vi "Command Pre-Buffer.vi"(2 "All Robot Commands In":T1, 3 "Startup":bool, 4 "Cmd Parameter 4":string, 5 "Cmd Parameter 3":dbl, 6 "Cmd Parameter 2":dbl, 7 "Cmd Parameter 1":dbl) -> (0 "All Robot Commands Out":T1, 1 "Completed":bool)   [LabVIEW 2016]
uses:
  Subsystems/All Robot Commands.ctl
  Subsystems/Drive and Climb SS/Drive + Climb Commands 2017.ctl
  Subsystems/Gear Delivery SS/Gear Delivery Commands.ctl
  Subsystems/Conveyor and Shooter SS/Conveyor and Shooter Commands.ctl
  Subsystems/Ball Intake SS/Ball Intake Commands.ctl
  Command Execution State.ctl
panel:
  # "Sample robot\ncontrol output.\nReplace with \nactual teleop \ncontrol signal \nstructure."
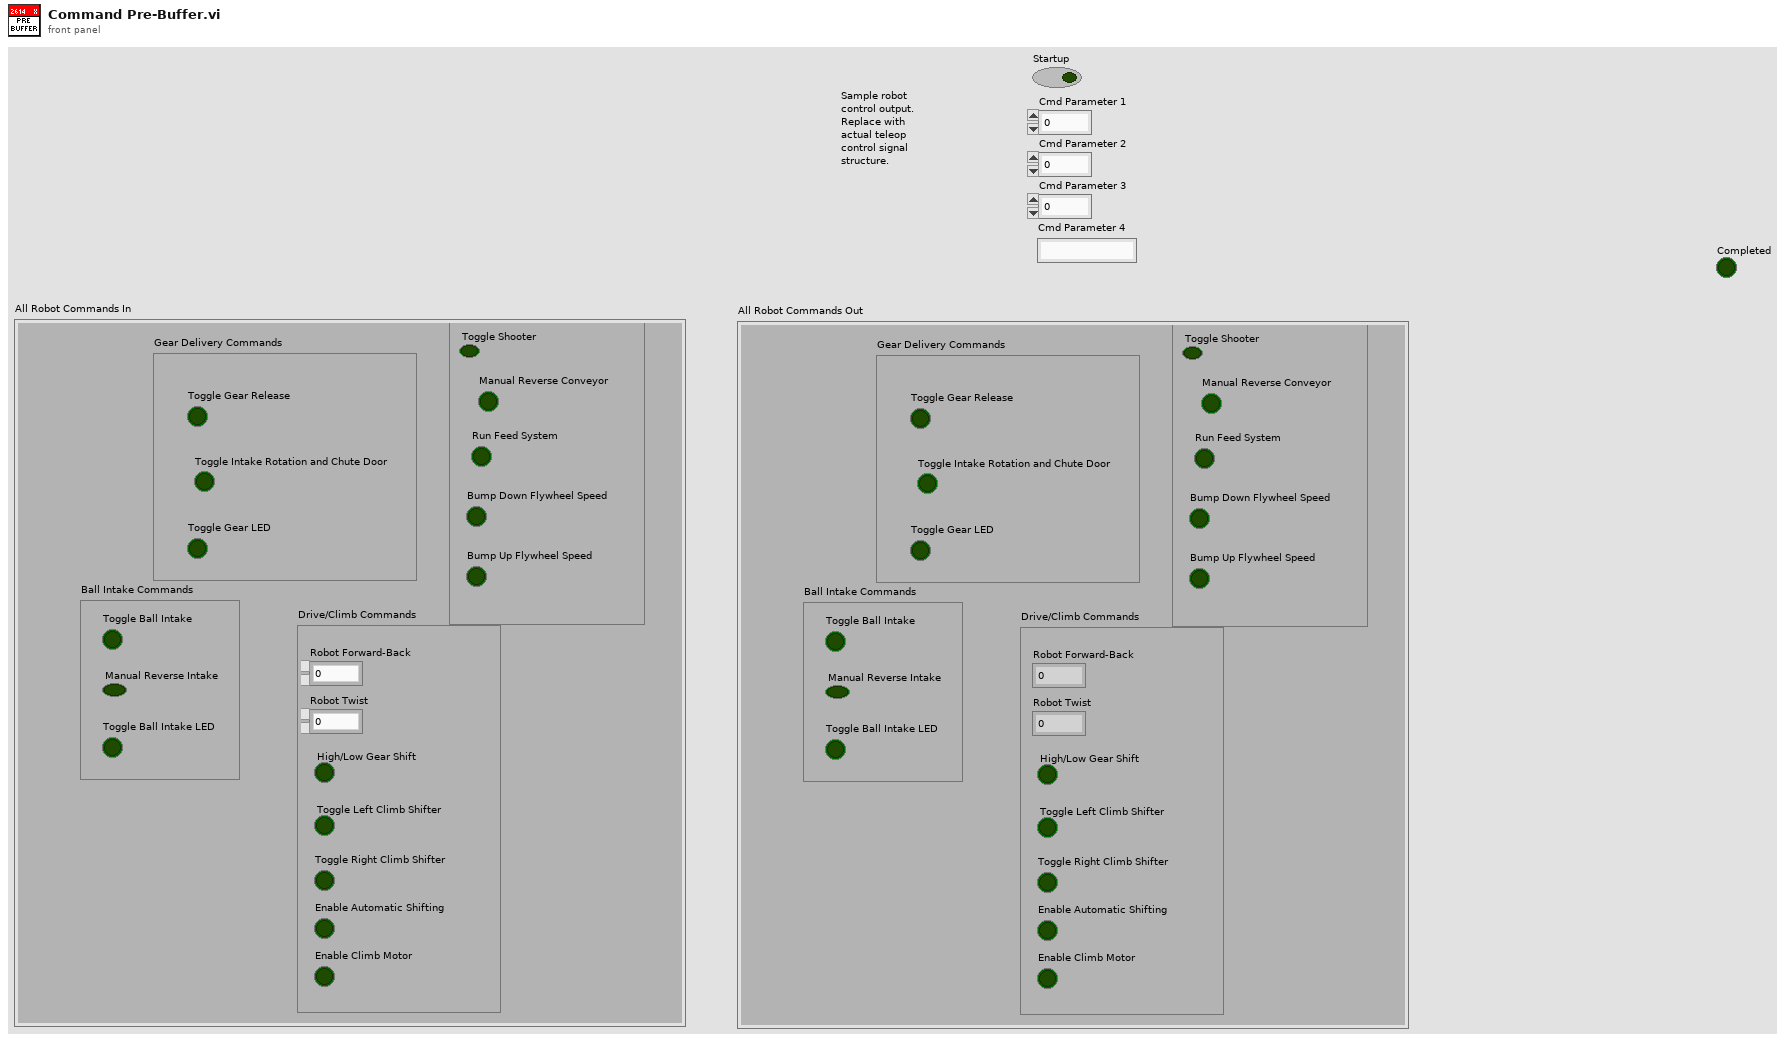
[diagram p1: front panel]
types:
  T1 = typedef "All Robot Commands.ctl" = cluster{"Drive/Climb Commands":T2, "Gear Delivery Commands":T3, "Shooter and Conveyor Commands":T4, "Ball Intake Commands":T5}
  T2 = typedef "Drive + Climb Commands 2017.ctl" = cluster{"Robot Forward-Back":dbl, "Robot Twist":dbl, "High/Low Gear Shift":bool, "Toggle Left Climb Shifter":bool, "Toggle Right Climb Shifter":bool, "Enable Automatic Shifting":bool, "Enable Climb Motor ":bool}
  T3 = typedef "Gear Delivery Commands.ctl" = cluster{"Toggle Gear Release":bool, "Toggle Intake Rotation and Chute Door":bool, "Toggle Gear LED":bool}
  T4 = typedef "Conveyor and Shooter Commands.ctl" = cluster{"Toggle Shooter":bool, "Manual Reverse Conveyor":bool, "Run Feed System":bool, "Bump Down Flywheel Speed":bool, "Bump Up Flywheel Speed":bool}
  T5 = typedef "Ball Intake Commands.ctl" = cluster{"Toggle Ball Intake":bool, "Manual Reverse Intake":bool, "Toggle Ball Intake LED":bool}
  T6 = typedef "Command Execution State.ctl" = enum16{"Initialize", "Execute", "Finish"}
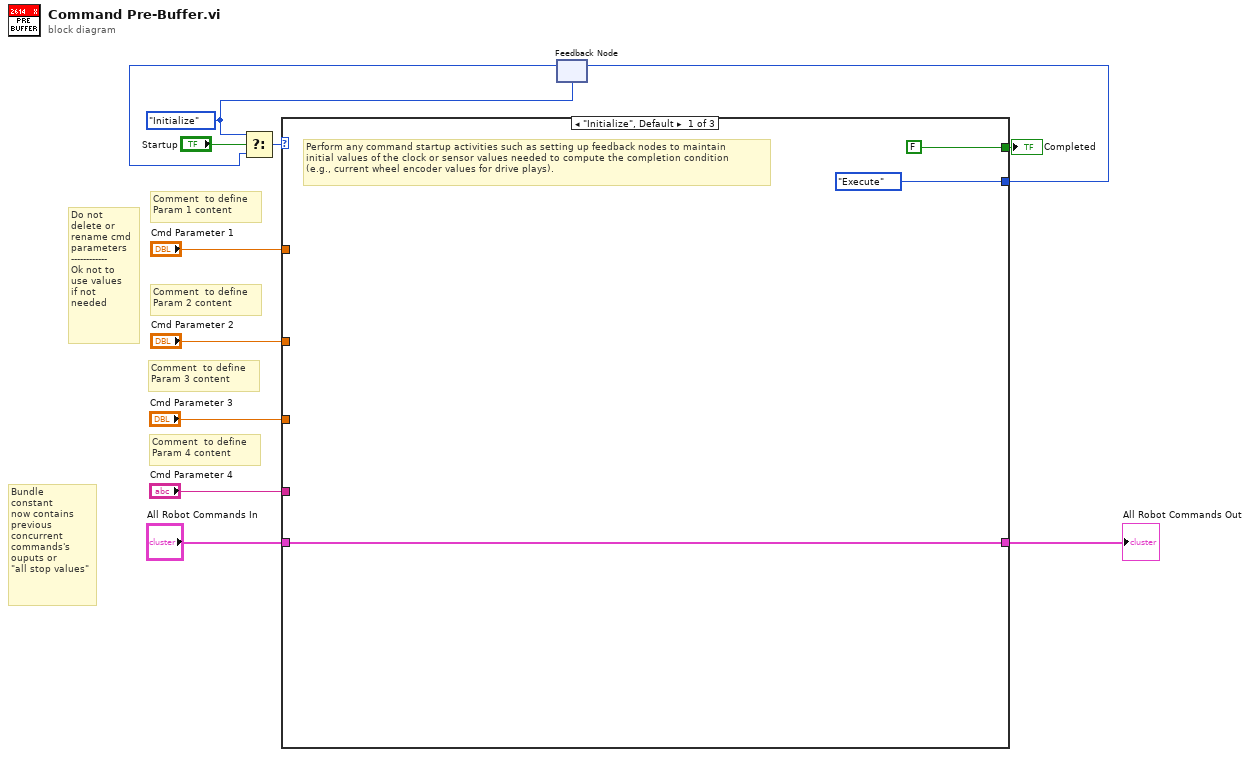
[diagram p0: block diagram]
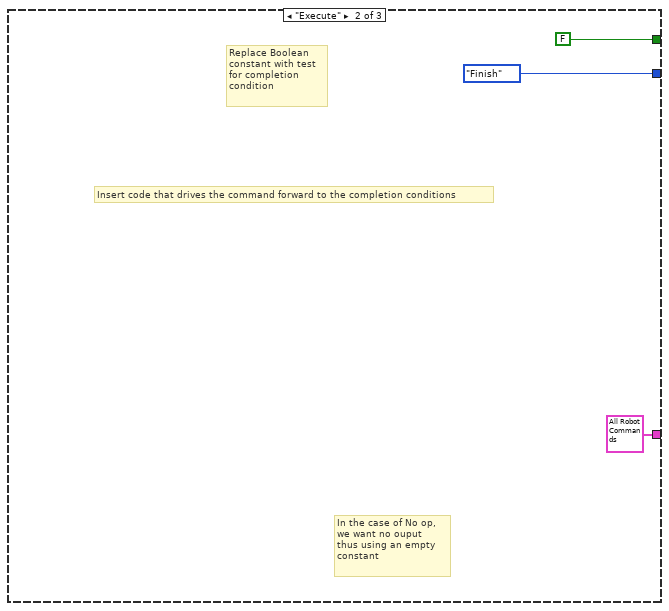
[diagram p2: hidden frame]
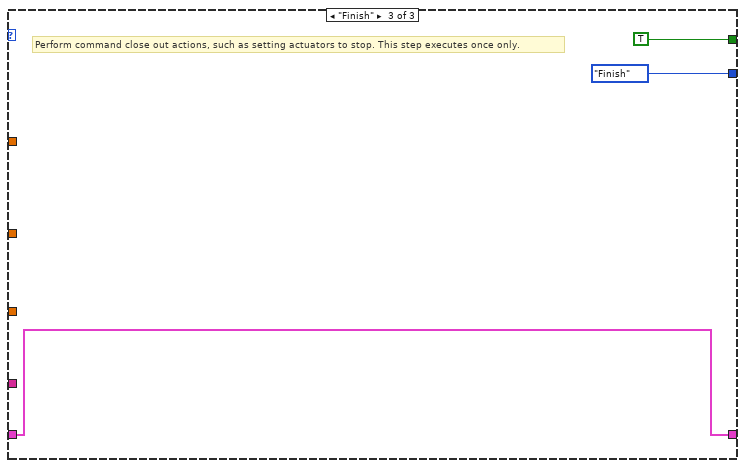
[diagram p3: hidden frame]
diagram:
  w7 = Command_Execution_State."Initialize" ("Play State")
  # "Comment  to define\nParam 4 content"
  # "Comment  to define\nParam 3 content"
  # "Bundle \nconstant\nnow contains\nprevious \nconcurrent\ncommands's\nouputs or\n\"all stop values\""
  # "Do not \ndelete or\nrename cmd\nparameters\n------------\nOk not to \nuse values\nif not \nneeded"
  # "Comment  to define\nParam 2 content"
  # "Comment  to define\nParam 1 content"
  n1 = feedback #1(w7) -> (w8:T6)
  n2 = Select(t=w7, s="Startup", f=w8) -> (s? t:f=w12:T6)
  n3 = case shown="\"Initialize\", Default" w12 {
    tunnel: [FALSE FALSE TRUE] -> w10
    tunnel: [Command_Execution_State."Execute" ("Play State") Command_Execution_State."Finish" ("Play State") Command_Execution_State."Finish" ("f")] -> w9
    tunnel: "Cmd Parameter 1" -> [_ _ _]
    tunnel: "Cmd Parameter 2" -> [_ _ _]
    tunnel: [w13 T1 {"Drive/Climb Commands"={"Robot Forward-Back"=0.0, "Robot Twist"=0.0, "High/Low Gear Shift"=FALSE, "Toggle Left Climb Shifter"=FALSE, "Toggle Right Climb Shifter"=FALSE, "Enable Automatic Shifting"=FALSE, "Enable Climb Motor "=FALSE}, "Gear Delivery Commands"={"Toggle Gear Release"=FALSE, "Toggle Intake Rotation and Chute Door"=FALSE, "Toggle Gear LED"=FALSE}, "Shooter and Conveyor Commands"={"Toggle Shooter"=FALSE, "Manual Reverse Conveyor"=FALSE, "Run Feed System"=FALSE, "Bump Down Flywheel Speed"=FALSE, "Bump Up Flywheel Speed"=FALSE}, "Ball Intake Commands"={"Toggle Ball Intake"=FALSE, "Manual Reverse Intake"=FALSE, "Toggle Ball Intake LED"=FALSE}} ("All Robot Commands") w19] -> w1
    tunnel: "All Robot Commands In" -> [w13 _ w19]
    tunnel: "Cmd Parameter 3" -> [_ _ _]
    tunnel: "Cmd Parameter 4" -> [_ _ _]
    frame "Initialize", Default {
      # "Perform any command startup activities such as setting up feedback nodes to maintain \ninitial values of the clock or sensor values needed to compute the completion condition\n(e.g., current wheel encoder values for drive plays)."
    }
    frame "Execute" {
      # "In the case of No op, \nwe want no ouput \nthus using an empty \nconstant"
      # "Replace Boolean\nconstant with test \nfor completion \ncondition"
      # "Insert code that drives the command forward to the completion conditions"
    }
    frame "Finish" {
      # "Perform command close out actions, such as setting actuators to stop. This step executes once only."
    }
  }
  "Completed" <- w10
  "All Robot Commands Out" <- w1
  n4 = feedback-in #1(w9) -> ()
